vi "OpenExtendedSession.vi"(8 "error in (no error)":errorcluster, 10 "SessionID":string, 11 "UDS Session Parameters":T1={"XNET Interface"="CAN1@nixnet", "BaudRate"=500000, "Transmit ID"=470077443, "Receive ID"=470073347} {"Receive ID" format="%x"; "Transmit ID" format="%x"}) -> (0 "error out":errorcluster)   [LabVIEW 2021, in "Lunar UDS CAN.lvlib"]
uses:
  Lunar UDS CAN.lvlib
  Controls/UDSSessionParameters.ctl
  Controls/UDSActions.ctl
  93d01b5f-7ffe-4e0a-9d16-9465dff62216.vi
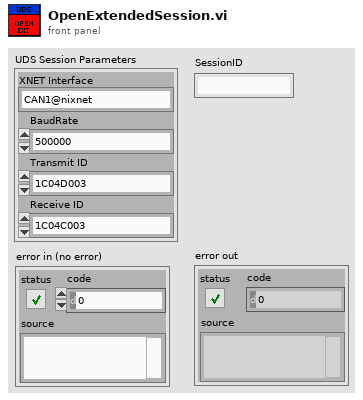
[diagram p1: front panel]
types:
  T1 = typedef "Lunar UDS CAN.lvlib/UDSSessionParameters.ctl" = cluster{"XNET Interface":string, "BaudRate":u64, "Transmit ID":i32, "Receive ID":i32}
  T2 = typedef "Lunar UDS CAN.lvlib/UDSActions.ctl" = enum16{"Open Session", "Connect To Diagnostic Session", "Send Tester Present", "ECU Reset", "Write String Data", "Write Byte Data", "Read Data", "Close Session", "Close All Sessions"}
  T3 = cluster{"Start Tester Present":bool, "Tester Present Period":dbl}
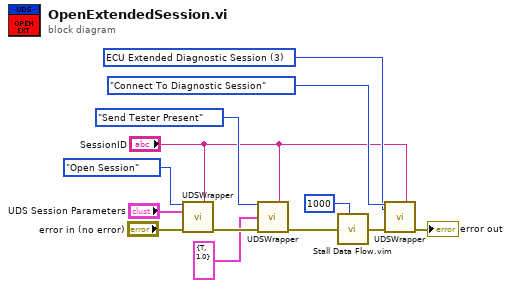
[diagram p0: block diagram]
diagram:
  w6 = u16 3 items=["Default Session"=1, "ECU Programming Session"=2, "ECU Extended Diagnostic Session"=3] ("Session Type")
  n1 = call "UDSWrapper.vi"("UDS Action"=UDSActions."Open Session", "SessionID"="SessionID", "UDS Session Parameters"="UDS Session Parameters", "error in (no error)"="error in (no error)") -> ("error out"=w11:errorcluster)  [unwired: 9 in, 2 out]
  n2 = call "UDSWrapper.vi"("UDS Action"=UDSActions."Send Tester Present", "SessionID"="SessionID", "Tester Present"=T3 {"Start Tester Present"=TRUE, "Tester Present Period"=1.0}, "error in (no error)"=w11) -> ("error out"=w8:errorcluster)  [unwired: 9 in, 2 out]
  n3 = call "Stall Data Flow.vim"("value in"=w8, "milliseconds to wait"=u32 1000) -> ("value out"=w3:errorcluster)  [unwired: 1 out]
  n4 = call "UDSWrapper.vi"("UDS Action"=UDSActions."Connect To Diagnostic Session", "Session Type"=w6, "SessionID"="SessionID", "error in (no error)"=w3) -> ("error out"=→"error out":errorcluster)  [unwired: 9 in, 2 out]
